vi "Write I8 Value.vi"(8 "error in (no error)":errorcluster, 10 "I8":i8, 11 "Numeric in":refnum<class "Abs_I16 Integer.lvclass">) -> (0 "error out":errorcluster, 3 "Numeric out":refnum<class "Abs_I16 Integer.lvclass">)   [LabVIEW 2021, in "Abs_I16 Integer.lvclass"]
uses:
  Abs_I16 Integer.lvclass
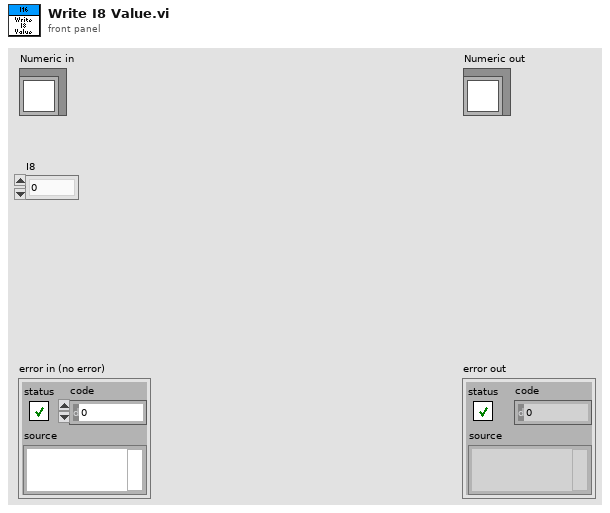
[diagram p1: front panel]
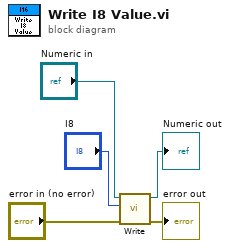
[diagram p0: block diagram]
diagram:
  n1 = call-dynamic "Write.vi"("error in (no error)"="error in (no error)", "Value"="I8", "Double Float.lvclass_340760 in"="Numeric in") -> ("error out"=→"error out":errorcluster, "Double Float.lvclass_340760 out"=→"Numeric out":refnum<class "Abs_I16 Integer.lvclass">)  [unwired: 7 in]
